vi "Program seq path.vi"(11 "Program sequence":string="data\\Featurelist.bin") -> (3 "File path":path)   [LabVIEW 2015]
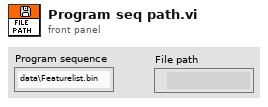
[diagram p1: front panel]
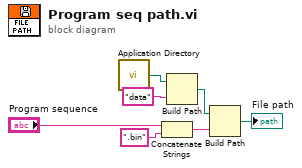
[diagram p0: block diagram]
diagram:
  n1 = call <vilib>:"Application Directory.vi"() -> ("Application Directory"=w1:path)
  n2 = Concatenate Strings("Program sequence", ".bin" ("string")) -> (w2:string)
  n3 = Build Path(base path=w1, name or relative path="data") -> (appended path=w5:path)
  n4 = Build Path(base path=w5, name or relative path=w2) -> (appended path=→"File path":path)
